vi "Launch Mag Lab Measure.vi"() -> ()   [LabVIEW 2015]
uses:
  MagLabMeasureApp/MagLabMeasureApp.lvclass
  <vilib>/ActorFramework/Actor/Actor.lvclass
panel:
  out "Error Out":errorcluster
  in  "Error In":errorcluster
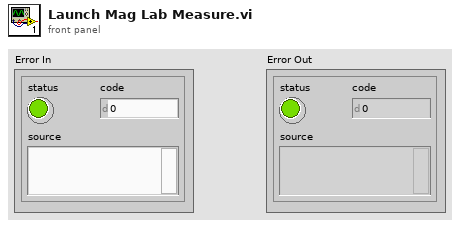
[diagram p1: front panel]
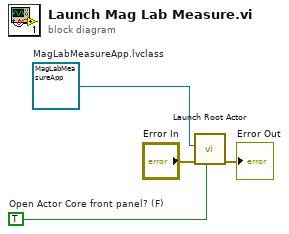
[diagram p0: block diagram]
diagram:
  w1 = TRUE  # Open Actor Core front panel? (F)
  w4 = refnum<class "MagLabMeasureApp.lvclass"> refnum  # MagLabMeasureApp.lvclass
  n1 = call <vilib>:"Launch Root Actor.vi"("Open Actor Core front panel? (F)"=w1, "error in (no error)"="Error In", "Actor"=w4) -> ("error out"=→"Error Out":errorcluster)  [unwired: 7 in, 1 out]
